vi "coil-set-current-slave.vi"(0 "GPIB adr in":string, 1 "Current (100% scale)":dbl min=0.0 max=10.0 step=0.01, 2 "current (1% scale)":sgl min=0 max=10 step=0.01) -> (20 "GPIB adr out":string, 27 "error out":errorcluster caption="sortie d'erreur" {"code" format="%.0x"})   [LabVIEW 2010]
doc: "Launches the Instrument I/O Assistant, which you can use to communicate with message-based instruments and graphically parse the response. For example you can communicate with an instrument that uses a serial, Ethernet, or GPIB interface."
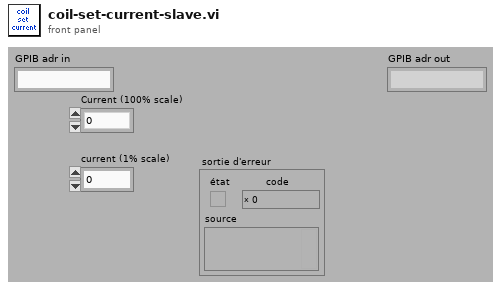
[diagram p1: front panel]
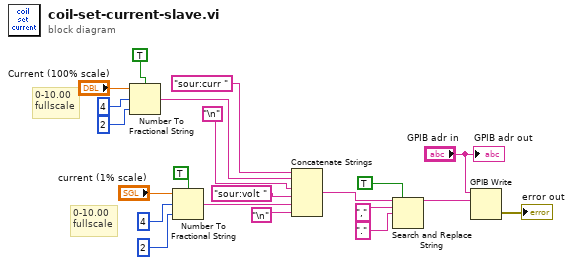
[diagram p0: block diagram]
diagram:
  # "0-10.00\nfullscale"
  # "0-10.00\nfullscale"
  n1 = Number To Fractional String(use system decimal point (T)=TRUE, number="Current (100% scale)", width (-)=i16 4, precision (6)=i16 2) -> (F-format string=w2:string)
  n2 = Number To Fractional String(use system decimal point (T)=TRUE, number="current (1% scale)", width (-)=i16 4, precision (6)=i16 2) -> (F-format string=w8:string)
  n3 = Concatenate Strings("sour:curr " ("staticText"), w2, "\n", "sour:volt " ("staticText"), w8, "\n") -> (w7:string)
  n4 = Search and Replace String(replace all?=TRUE ("replace all? (F)"), input string=w7, search string=",", replace string="." ("replace string (\"\")")) -> (result string=w4:string)  [unwired: 1 in, 6 out]
  n5 = GPIB Write(0:"GPIB adr in", 1:w4) -> (6:→"error out":errorcluster)  [unwired: 1 in, 3 out]
  "GPIB adr out" <- "GPIB adr in"
